vi "多点图.vi"() -> ()   [LabVIEW 2018]
panel:
  in  "停止":bool
  in  "滑动杆":dbl(slide) scale=0.0..900.0
  out "波形图":dbl[](graph)
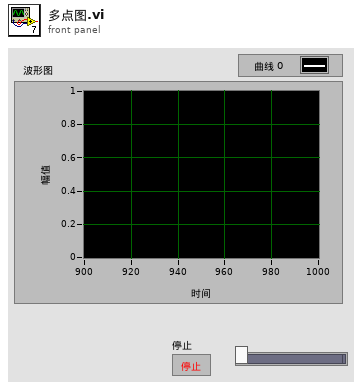
[diagram p1: front panel]
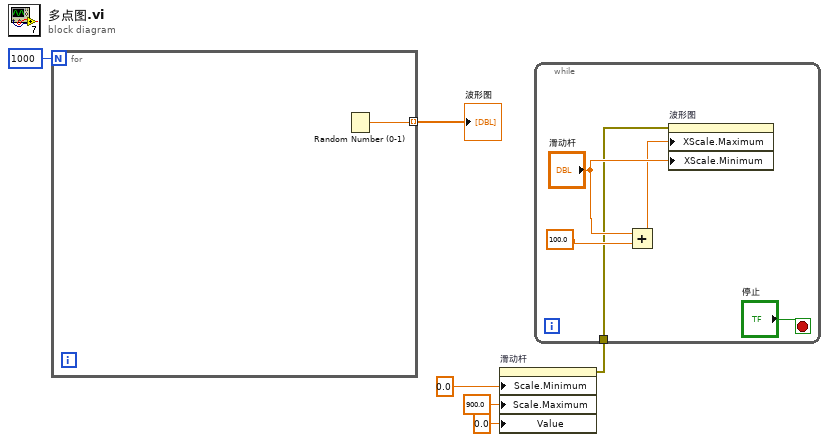
[diagram p0: block diagram]
diagram:
  n1 = for {
    N: 1000 -> [_]
    tunnel: [w7] -> w5 mode=indexing
    n2 = Random Number (0-1)() -> (number: 0 to 1=w7:dbl)
  }
  "波形图" <- w5
  n3 = property on="滑动杆" class="Slide (严格)"("Scale.Minimum"=0.0 ("标尺.范围:最小值"), "Scale.Maximum"=900.0 ("标尺.范围:最大值"), "Value"=0.0 ("滑动杆")) -> (error out=w1:errorcluster)  [unwired: 2 in, 1 out]
  n4 = while {
    tunnel: w1 -> [w8]
    stop <- "停止" stop-if-true
    n5 = Add(x="滑动杆", y=100.0) -> (x+y=w10:dbl)
    n6 = property on="波形图" class="WFGraph (严格)"(error in=w8, "XScale.Maximum"=w10, "XScale.Minimum"="滑动杆") -> ()  [unwired: 1 in, 2 out]
  }
